vi "OPC UA Server_String_Secure.vi"() -> ()   [LabVIEW 2017]
uses:
  <vilib>/OPCUA/controls/Data Type.ctl
  <vilib>/OPCUA/controls/Supported Security Policies.ctl
  <vilib>/OPCUA/NI OPC UA Server.lvlib
  <vilib>/OPCUA/NI OPC UA Utility.lvlib
panel:
  out "temp node ID":string
  in  "stop":bool
  out "error out":errorcluster
  out "message node ID":string
  out "server endpoint URL":string
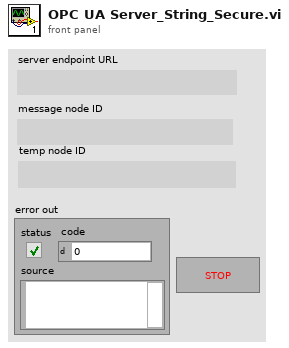
[diagram p1: front panel]
types:
  T1 = typedef "Data Type.ctl" = u16
  T2 = cluster{"name":string, "data type":T1, "access level":u16, "description":string}
  T3 = typedef "Supported Security Policies.ctl" = cluster{"None":bool, "Sign with Basic128Rsa15":bool, "Sign and Encrypt with Basic128Rsa15":bool, "Sign with Basic256":bool, "Sign and Encrypt with Basic256":bool}
  T4 = typedef "OPC UA Server Refnum.ctl" = refnum<k21>
  T5 = typedef "NodeId.ctl" = string
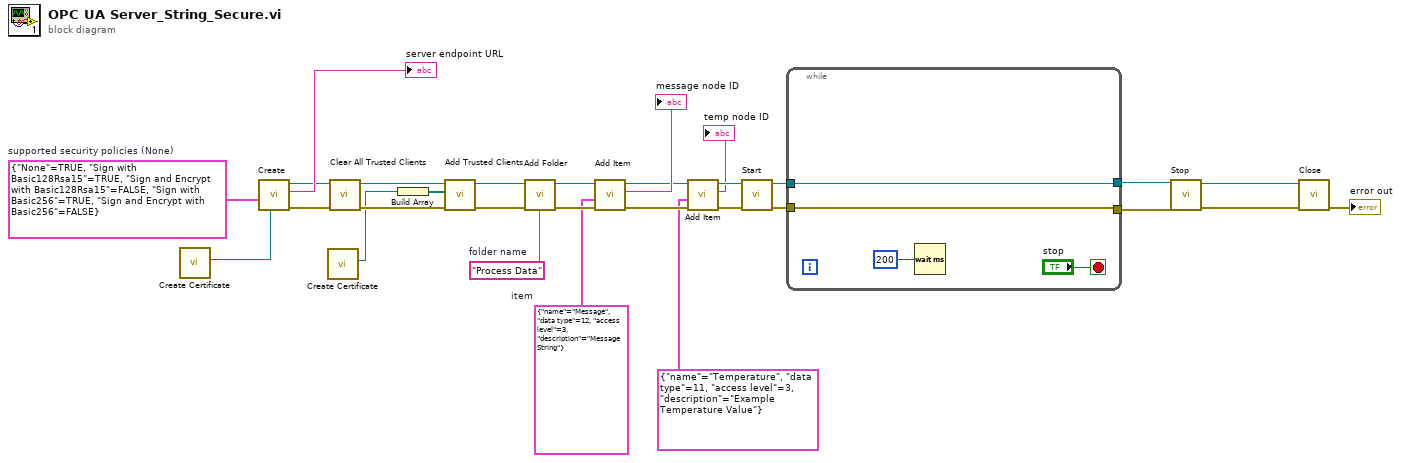
[diagram p0: block diagram]
diagram:
  w16 = T3 {"None"=TRUE, "Sign with Basic128Rsa15"=TRUE, "Sign and Encrypt with Basic128Rsa15"=FALSE, "Sign with Basic256"=TRUE, "Sign and Encrypt with Basic256"=FALSE}  # supported security policies (None)
  w25 = T2 {"name"="Message", "data type"=12, "access level"=3, "description"="Message String"}  # item
  w26 = "Process Data"  # folder name
  n1 = call <vilib>:"Create Certificate.vi"() -> ("certificate path"=w9:path)  [unwired: 8 in, 3 out]
  n2 = call <vilib>:"Create.vi"("server certificate file"=w9, "supported security policies (None)"=w16) -> ("error out"=w12:errorcluster, "server endpoint URL"=→"server endpoint URL":string, "OPC UA server refnum out"=w13:T4)  [unwired: 7 in]
  n3 = call <vilib>:"Create Certificate.vi"() -> ("certificate path"=w8:path)  [unwired: 8 in, 3 out]
  n4 = call <vilib>:"Clear All Trusted Clients.vi"("error in (no error)"=w12, "OPC UA server refnum in"=w13) -> ("error out"=w14:errorcluster, "OPC UA server refnum out"=w15:T4)  [unwired: 8 in]
  n5 = Build Array(w8) -> (w7:path[])
  n6 = call <vilib>:"Add Trusted Clients.vi"("error in (no error)"=w14, "trusted client certificates"=w7, "OPC UA server refnum in"=w15) -> ("error out"=w10:errorcluster, "OPC UA server refnum out"=w11:T4)  [unwired: 7 in]
  n7 = call <vilib>:"Add Folder.vi"("error in (no error)"=w10, "folder name"=w26, "OPC UA server refnum in"=w11) -> ("error out"=w28:errorcluster, "OPC UA server refnum out"=w29:T4)  [unwired: 5 in, 1 out]
  n8 = call <vilib>:"Add Item.vi"("error in (no error)"=w28, "item"=w25, "OPC UA server refnum in"=w29) -> ("error out"=w5:errorcluster, "item node ID"=→"message node ID":T5, "OPC UA server refnum out"=w6:T4)  [unwired: 4 in, 1 out]
  n9 = call <vilib>:"Add Item.vi"("error in (no error)"=w5, "item"=T2 {"name"="Temperature", "data type"=11, "access level"=3, "description"="Example Temperature Value"}, "OPC UA server refnum in"=w6) -> ("error out"=w4:errorcluster, "item node ID"=→"temp node ID":T5, "OPC UA server refnum out"=w3:T4)  [unwired: 4 in, 1 out]
  n10 = call <vilib>:"Start.vi"("error in (no error)"=w4, "OPC UA server refnum in"=w3) -> ("error out"=w22:errorcluster, "OPC UA server refnum out"=w23:T4)  [unwired: 7 in, 1 out]
  n11 = while {
    tunnel: [w33] -> w20
    tunnel: w23 -> [w33]
    tunnel: [w32] -> w21
    tunnel: w22 -> [w32]
    stop <- "stop" stop-if-true
    n12 = Wait (ms)(milliseconds to wait=u32 200) -> ()  [unwired: 1 out]
  }
  n13 = call <vilib>:"Stop.vi"("error in (no error)"=w21, "OPC UA server refnum in"=w20) -> ("error out"=w18:errorcluster, "OPC UA server refnum out"=w19:T4)  [unwired: 8 in]
  n14 = call <vilib>:"Close.vi"("error in (no error)"=w18, "OPC UA server refnum in"=w19) -> ("error out"=→"error out":errorcluster)  [unwired: 9 in]
